vi "TiffToJpeg.vi"() -> ()   [LabVIEW 2009]
panel:
  out "KONIEC":bool
  out "error out":errorcluster
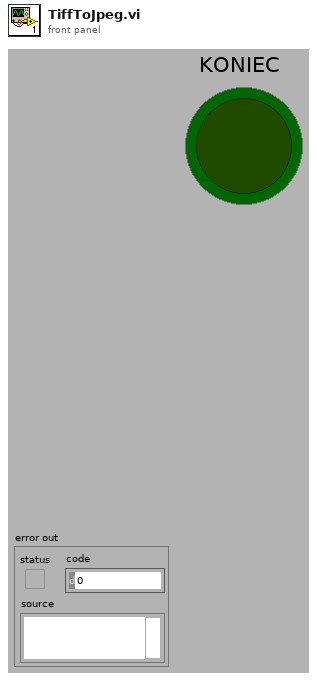
[diagram p1: front panel]
types:
  T1 = typedef "Image Type" = u32
  T2 = typedef "IMAQ Image.ctl" = refnum<image>
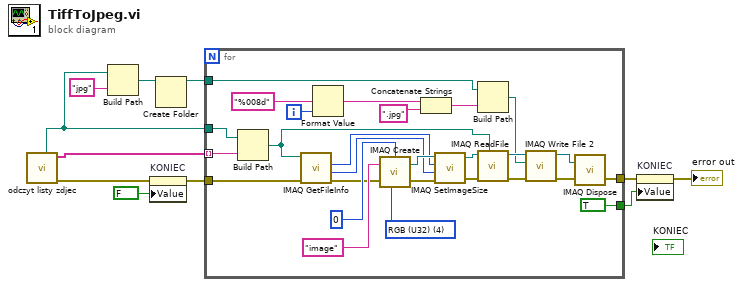
[diagram p0: block diagram]
diagram:
  n1 = call "odczyt listy zdjec.vi"() -> ("error out"=w5:errorcluster, "lista zdjec"=w11:string[], "sciezka do zdjec"=w7:path)  [unwired: 1 in, 3 out]
  n2 = Build Path(base path=w7, name or relative path="jpg") -> (appended path=w8:path)
  n3 = property on="KONIEC" class="Bool (strict)"(error in=w5, "Value"=FALSE) -> (error out=w4:errorcluster)  [unwired: 1 in, 1 out]
  n4 = Create Folder(path (use dialog)=w8) -> (created path=w9:path)  [unwired: 2 in, 2 out]
  n5 = for {
    tunnel: w7 -> [w28]
    tunnel: w4 -> [w27]
    tunnel: [w23] -> w3
    tunnel: w11 -> [w21] mode=indexing
    tunnel: w9 -> [w16]
    tunnel: [TRUE] -> w1
    i -> [w14]
    w12 = T1 4 items=["Grayscale (U8)", "Grayscale (I16)", "Grayscale (SGL)", "Complex (CSG)", "RGB (U32)", "HSL (U32)", "RGB (U64)", "Grayscale (U16)"] ("Image Type")
    n6 = Build Path(base path=w28, name or relative path=w21) -> (appended path=w38:path)
    n7 = call "IMAQ GetFileInfo"("error in (no error)"=w27, "File Path"=w38) -> ("error out"=w31:errorcluster, "Y Resolution"=w32:i32, "X Resolution"=w33:i32)  [unwired: 3 in, 4 out]
    n8 = Format Value(format string="%008d", value (0)=w14) -> (output string=w20:string)  [unwired: 1 in]
    n9 = call "IMAQ Create"("Border Size"=0, "Image Name"="image", "Image Type"=w12, "error in (no error)"=w31) -> ("New Image"=w35:T2, "error out"=w30:errorcluster)  [unwired: 1 in]
    n10 = Concatenate Strings(w20, ".jpg" ("string")) -> (w17:string)
    n11 = call "IMAQ SetImageSize"("error in (no error)"=w30, "Y Resolution"=w32, "X Resolution"=w33, "Image"=w35) -> ("error out"=w29:errorcluster, "Image Out"=w34:T2)  [unwired: 1 in]
    n12 = Build Path(base path=w16, name or relative path=w17) -> (appended path=w15:path)
    n13 = call "IMAQ ReadFile"("File Path"=w38, "error in (no error)"=w29, "Image"=w34) -> ("error out"=w22:errorcluster, "Image Out"=w26:T2)  [unwired: 4 in, 3 out]
    n14 = call-poly "IMAQ Write File 2"("error in (no error)"=w22, "File Path"=w15, "Image"=w26) -> ("error out"=w24:errorcluster, "Image Out (duplicate)"=w25:T2)  [unwired: 7 in]
    n15 = call "IMAQ Dispose"("Image"=w25, "error in (no error)"=w24) -> ("error out"=w23:errorcluster)  [unwired: 4 in]
  }
  n16 = property on="KONIEC" class="Bool (strict)"(error in=w3, "Value"=w1) -> (error out=→"error out":errorcluster)  [unwired: 1 in, 1 out]
